vi "GV stage strigger duration.vi"() -> ()   [LabVIEW 2017]
panel:
  out "StageTriggerDuration_tick":u16
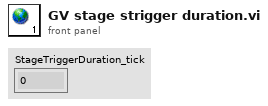
[diagram p1: front panel]
diagram:
